vi "Picometer Control_i.vi"(0 "Cmd":u8 format="%.0x", 2 "execute":bool, 5 "ulValue":u32, 7 "uLPtr":u32[](array[numeric]), 9 "BytePtr":u8[](array[numeric]), 11 "error in (no error)":errorcluster) -> (4 "function return":string, 6 "ulValue":u32, 8 "uLPtr":u32[](array[numeric]), 10 "BytePtr":u8[](array[numeric]), 15 "error out":errorcluster)   [LabVIEW 2017, in "ZBOX_IS.lvlib"]
doc: "char *PicometerControl(\n unsigned char Cmd, unsigned long ulValue, unsigned long *uLPtr, unsigned char *BytePtr );"
uses:
  ZBOX_IS.lvlib
  PicometerCtrl.dll
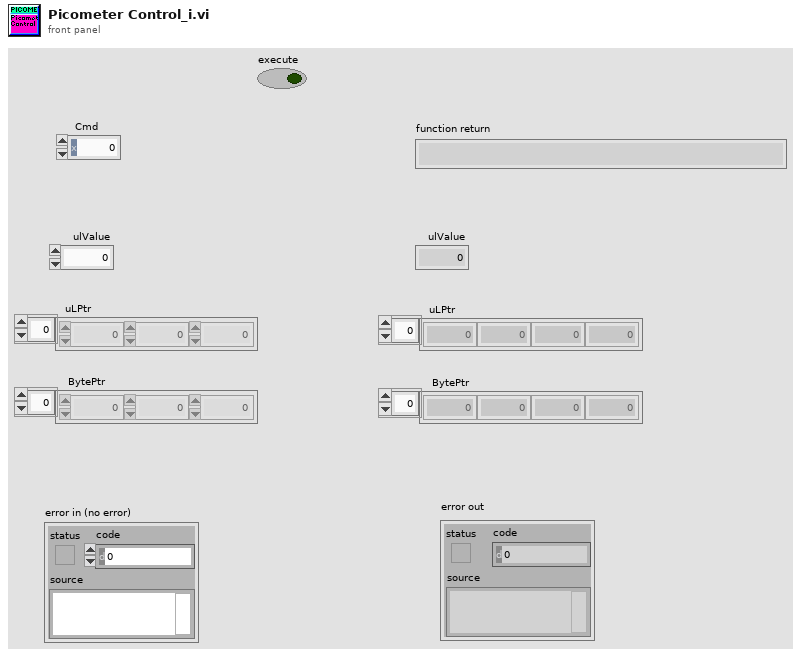
[diagram p1: front panel]
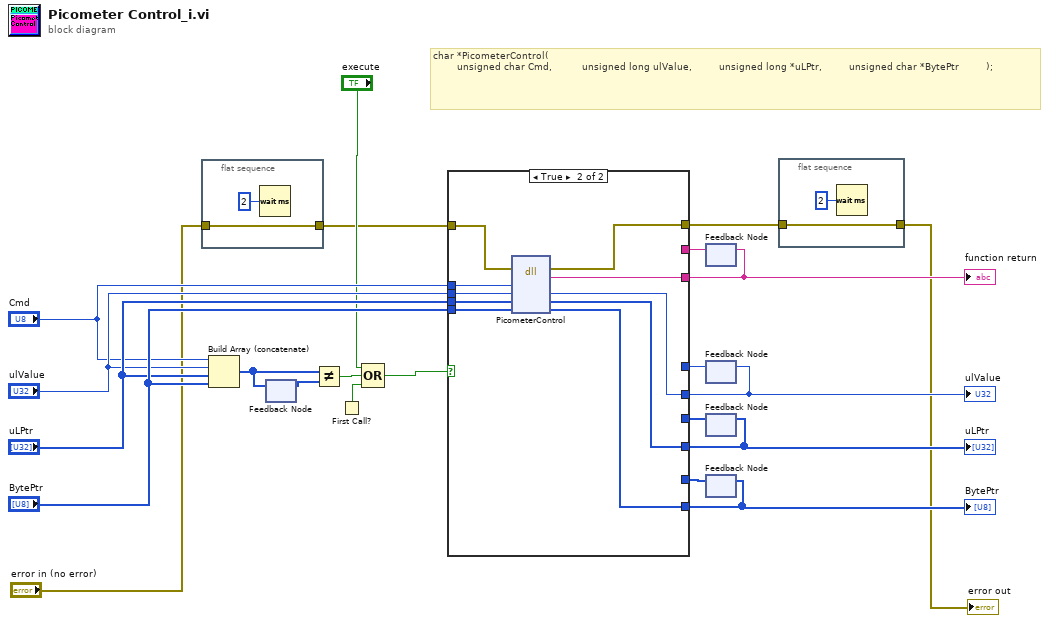
[diagram p0: block diagram]
diagram:
  # "char *PicometerControl(\n\t\t\t\t\t   unsigned char Cmd,\t\t\t\t\t\t\t   unsigned long ulValue,\t\t\t\t\t\t   unsigned long *uLPtr,\t\t\t\t\t\t   unsigned char *BytePtr\t\t\t\t\t\t   );"
  n1 = flat-sequence {
    tunnel: "error in (no error)" -> [w24]
    tunnel: [w24] -> w4
    frame #0 {
      n2 = Wait (ms)(milliseconds to wait=u32 2) -> ()  [unwired: 1 out]
    }
  }
  n3 = Build Array (concatenate)("Cmd", "ulValue", "uLPtr", "BytePtr") -> (w18:u32[])
  n4 = feedback-in #1(w18) -> ()
  n5 = feedback #1() -> (w17:u32[])  [unwired: 1 in]
  n6 = Not Equal?(x=w18, y=w17) -> (x != y?=w8:bool)
  n7 = First Call?() -> (First Call?: T/F=w1:bool)
  n8 = Compound Arithmetic op=OR("execute", w8, w1) -> (w2:bool)
  n9 = feedback #2() -> (w12:string)  [unwired: 1 in]
  n10 = feedback #3() -> (w11:u32)  [unwired: 1 in]
  n11 = feedback #4() -> (w10:u32[])  [unwired: 1 in]
  n12 = feedback #5() -> (w9:u8[])  [unwired: 1 in]
  n13 = case shown="True" w2 {
    tunnel: [w25 w39] -> w13
    tunnel: "Cmd" -> [_ w30]
    tunnel: "ulValue" -> [_ w38]
    tunnel: w4 -> [w26 w37]
    tunnel: [w26 w36] -> w6
    tunnel: "BytePtr" -> [_ w35]
    tunnel: [w27 w34] -> w16
    tunnel: "uLPtr" -> [_ w33]
    tunnel: [w28 w32] -> w15
    tunnel: [w29 w31] -> w14
    tunnel: w12 -> [w25 _]
    tunnel: w11 -> [w29 _]
    tunnel: w10 -> [w28 _]
    tunnel: w9 -> [w27 _]
    frame False {
    }
    frame True {
      n14 = dll-call lib="C:/Users/Marek/Desktop/Quadra Software Package v1.1/LabView/Zbox_is/Public/Configure/Low Level/__DLL_functions/PicometerCtrl.dll" fn="PicometerControl"(error in=w37, "Cmd"=w30, "ulValue"=w38, "uLPtr"=w33, "BytePtr"=w35) -> (error out=w36:errorcluster, "return type"=w39:string, "ulValue"=w31:u32, "uLPtr"=w32:u32[], "BytePtr"=w34:u8[])  [unwired: 3 in, 1 out]
    }
  }
  "function return" <- w13
  "ulValue" <- w14
  "BytePtr" <- w16
  "uLPtr" <- w15
  n15 = feedback-in #2(w13) -> ()
  n16 = feedback-in #3(w14) -> ()
  n17 = feedback-in #4(w15) -> ()
  n18 = feedback-in #5(w16) -> ()
  n19 = flat-sequence {
    tunnel: w6 -> [w41]
    tunnel: [w41] -> w5
    frame #0 {
      n20 = Wait (ms)(milliseconds to wait=u32 2) -> ()  [unwired: 1 out]
    }
  }
  "error out" <- w5
